vi "halve.vi"(1 "x":i16) -> (0 "y":i16)   [LabVIEW 2018, in "posit.lvlib"]
uses:
  posit.lvlib
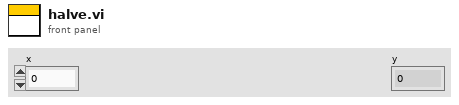
[diagram p1: front panel]
types:
  T1 = typedef "posit.lvlib/unpacked.ctl" = cluster{"sign":bool, "regime":i16, "exoinent":i16, "fraction":i16, "type":T2}
  T2 = typedef "posit.lvlib/specialnumber.ctl" = enum16{"Zero", "Regular", "NaN", "Infinity"}
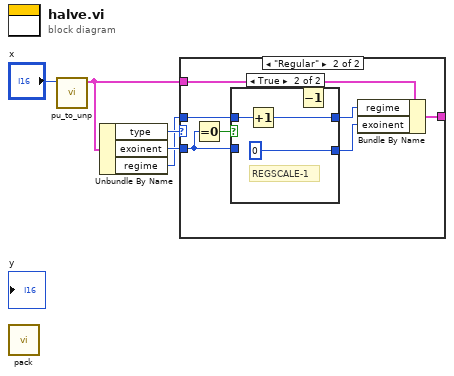
[diagram p0: block diagram]
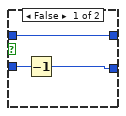
[diagram p3: hidden frame]
diagram:
  n1 = call "pack.vi"() -> ()  [unwired: 12 in]
  n2 = call "pu_to_unp.vi"("x"="x") -> ("y"=w1:T1)  [unwired: 10 in]
  n3 = Unbundle By Name(w1) -> ("type"=w4:T2, "exoinent"=w3:i16, "regime"=w2:i16)
  n4 = case shown="\"Regular\"" w4 {
    tunnel: w3 -> [_ w12]
    tunnel: w2 -> [_ w13]
    tunnel: w1 -> [w6 w11]
    tunnel: [w6 w10] -> _
    frame "Zero", Default {
    }
    frame "Regular" {
      n5 = Equal To 0?(x=w12) -> (x = 0?=w7:bool)
      n6 = case shown="True" w7 {
        tunnel: w13 -> [w14 w19]
        tunnel: w12 -> [w16 _]
        tunnel: [w15 i16 0] -> w8
        tunnel: [w14 w18] -> w9
        frame False {
          n7 = Decrement(x=w16) -> (x-1=w15:i16)
        }
        frame True {
          # "REGSCALE-1"
          n8 = Increment(x=w19) -> (x+1=w18:i16)
        }
      }
      n9 = Decrement() -> ()  [unwired: 1 in, 1 out]
      n10 = Bundle By Name(cluster=w11, "regime"=w9, "exoinent"=w8) -> (w10:T1)
    }
  }
